vi "create.vi"(11 "Message Enqueuer":refnum<class "Message Enqueuer.lvclass">) -> (3 "actor reporter":refnum<class "actor reporter.lvclass">)   [LabVIEW 2013, in "actor reporter.lvclass"]
uses:
  actor reporter.lvclass
  <vilib>/ActorFramework/Message Enqueuer/Message Enqueuer.lvclass
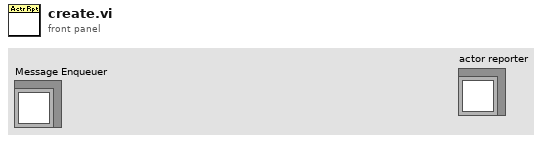
[diagram p1: front panel]
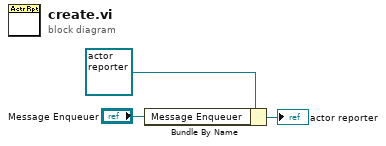
[diagram p0: block diagram]
diagram:
  n1 = Bundle By Name(cluster=refnum<class "actor reporter.lvclass"> refnum ("actor reporter in"), "Message Enqueuer"="Message Enqueuer") -> (→"actor reporter":refnum<class "actor reporter.lvclass">)
